vi "Firing Arm.vi"(11 "Input":bool) -> (0 "error out":errorcluster)   [LabVIEW 2012]
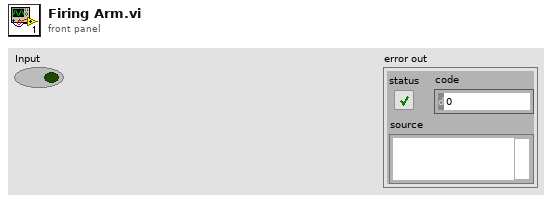
[diagram p1: front panel]
types:
  T1 = typedef "WPI_MotorControlDeviceRef.ctl" = cluster{"DeviceStatus":errorcluster, "Type":enum16{"PWM", "CAN"}, "PWM":cluster{"Digital Module":T2, "PWM Channel":T3, "DeadBand":T4}, "CAN":cluster{"Device Number":u8, "Control Mode":T5, "Semaphore":T6, "Max Vout":dbl}, "Invert":bool, "TransformRef":T7, "InvTransformRef":T7}
  T2 = typedef "FPGA_TypedefDigitalModule.ctl" = enum16{"Digital Module 1", "Digital Module 2"}
  T3 = typedef "FPGA_DIOPWMChannel.ctl" = enum8{"PWM 1", "PWM 2", "PWM 3", "PWM 4", "PWM 5", "PWM 6", "PWM 7", "PWM 8", "PWM 9", "PWM 10", "Invalid"}
  T4 = typedef "WPI_PWMDeadband.ctl" = cluster{"Name":string, "maxPositivePwm":i32, "minPositivePwm":i32, "centerPwm":i32, "maxNegativePwm":i32, "minNegativePwm":i32, "angularRange":u16}
  T5 = typedef "WPI_CANJaguar_ControlMode.ctl" = enum8{"Percent VBus", "Current", "Speed", "Position", "Voltage"}
  T6 = typedef "Semaphore RefNum" = refnum<k1>
  T7 = typedef "WPI_PWMTransform_ConPane.ctl" = refnum<vi>
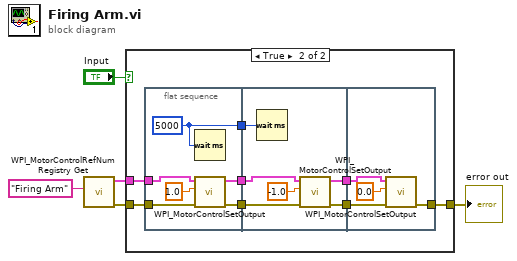
[diagram p0: block diagram]
diagram:
  n1 = call <vilib>:"WPI_MotorControlRefNum Registry Get.vi"("refnum name"="Firing Arm") -> ("error out"=w2:errorcluster, "MotorControlDevRef"=w5:T1)  [unwired: 9 in]
  n2 = case shown="True" "Input" {
    tunnel: w5 -> [_ w14]
    tunnel: w2 -> [w6 w10]
    tunnel: [w6 w7] -> w1
    frame False {
    }
    frame True {
      n3 = flat-sequence {
        tunnel: w14 -> [w19]
        tunnel: [w18] -> w13
        tunnel: [w17] -> w11
        tunnel: w10 -> [w16]
        tunnel: [w15] -> w9
        tunnel: w13 -> [w25]
        tunnel: [w24] -> w12
        tunnel: w11 -> [w23]
        tunnel: w9 -> [w22]
        tunnel: [w21] -> w8
        tunnel: w12 -> [w29]
        tunnel: w8 -> [w28]
        tunnel: [w27] -> w7
        frame #0 {
          w17 = u32 5000 ("milliseconds to wait")
          n4 = Wait (ms)(milliseconds to wait=w17) -> ()  [unwired: 1 out]
          n5 = call <vilib>:"WPI_MotorControlSetOutput.vi"("error in (no error)"=w16, "Output"=1.0, "MotorControlDevRef"=w19) -> ("error out"=w15:errorcluster, "MotorControlDevRef"=w18:T1)  [unwired: 6 in, 1 out]
        }
        frame #1 {
          n6 = Wait (ms)(milliseconds to wait=w23) -> ()  [unwired: 1 out]
          n7 = call <vilib>:"WPI_MotorControlSetOutput.vi"("error in (no error)"=w22, "Output"=-1.0, "MotorControlDevRef"=w25) -> ("error out"=w21:errorcluster, "MotorControlDevRef"=w24:T1)  [unwired: 6 in, 1 out]
        }
        frame #2 {
          n8 = call <vilib>:"WPI_MotorControlSetOutput.vi"("error in (no error)"=w28, "Output"=0.0, "MotorControlDevRef"=w29) -> ("error out"=w27:errorcluster)  [unwired: 6 in, 2 out]
        }
      }
    }
  }
  "error out" <- w1
